vi "Set Cookie Name.vi"(8 "error in (no error)":errorcluster, 10 "Cookie Name":string, 11 "Session in":refnum<class "Session.lvclass">) -> (0 "error out":errorcluster, 3 "Session out":refnum<class "Session.lvclass">)   [LabVIEW 2020, in "HTTP Server.lvlib" / "Session.lvclass"]
uses:
  Session.lvclass
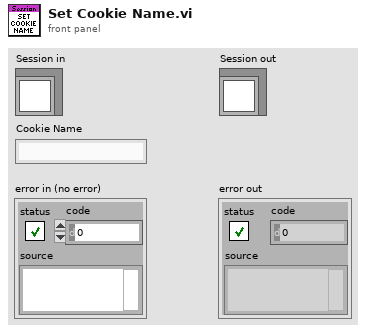
[diagram p1: front panel]
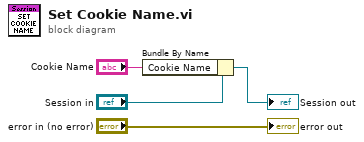
[diagram p0: block diagram]
diagram:
  n1 = Bundle By Name(cluster="Session in", "Cookie Name"="Cookie Name") -> (→"Session out":refnum<class "Session.lvclass">)
  "error out" <- "error in (no error)"
